vi "Set Dependency.vi"(8 "error in (no error)":errorcluster, 10 "Dependency":T1, 11 "LogEngine":refnum<class "LogEngine.lvclass">) -> (0 "error out":errorcluster, 3 "LogEngine out":refnum<class "LogEngine.lvclass">)   [LabVIEW 2022 SP3, in "LogEngine.lvclass"]
doc: "Developed by Kevin Thompson\nkevin@thompsonengineering.net\n\nCopyright 2018-2020\nThompson Engineering, LLC"
uses:
  LogEngine.lvclass
  LogEngine.lvclass/LogEngine.ctl
  Support/DataQueues/DataQueues.lvclass
  DAQ/DAQ.lvclass
  Data Types/Dependency--cluster.ctl
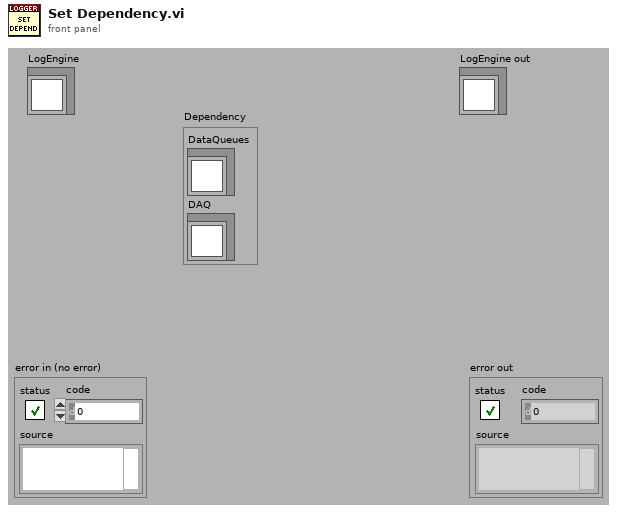
[diagram p1: front panel]
types:
  T1 = typedef "LogEngine.lvclass/Dependency--cluster.ctl" = cluster{"DataQueues":refnum<class "DataQueues.lvclass">, "DAQ":refnum<class "DAQ.lvclass">}
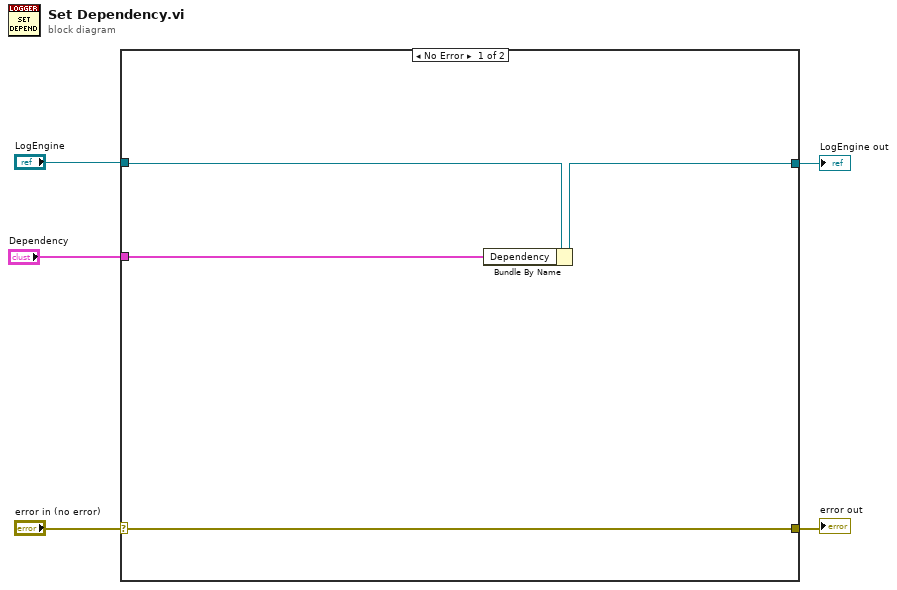
[diagram p0: block diagram]
diagram:
  n1 = case shown="No Error" "error in (no error)" {
    selector: "error in (no error)" -> [w8 w11]
    tunnel: [w8 w11] -> w4
    tunnel: [w6 w10] -> w2
    tunnel: "LogEngine" -> [w7 w10]
    tunnel: "Dependency" -> [w9 _]
    frame No Error {
      n2 = Bundle By Name(cluster=w7, "Dependency"=w9) -> (w6:refnum<class "LogEngine.lvclass">)
    }
    frame Error {
    }
  }
  "error out" <- w4
  "LogEngine out" <- w2
